vi "Read 1 Swipe X Z Vector.vi"(8 "Error In":errorcluster, 11 "Leap Handle":T2) -> (0 "Error Out":errorcluster, 1 "Gesture State":T1, 2 "XZ Swipe Vector":cluster{"X Direction":sgl, "Z Direction":sgl}, 3 "Leap Handle":T2)   [LabVIEW 2011, in "LVH-Leap.lvlib"]
uses:
  LVH-Leap.lvlib
  Private/Type Defs/Leap Handle.ctl
  C:/github/labviewhacker/LVH-Leap/LabVIEW/vi.lib/LabVIEW Hacker/Leap/Private/Libs/LeapCSharp.NET3.5.dll
  Private/Libs/LeapCSharp.NET3.5.dll
  Private/Type Defs/Gesture State.ctl
  Read 1 Swipe.vi
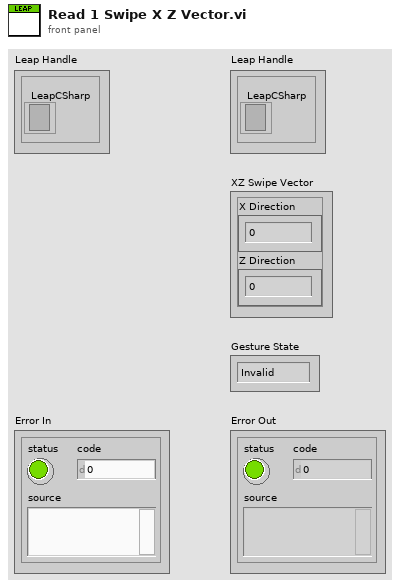
[diagram p1: front panel]
types:
  T1 = typedef "LVH-Leap.lvlib/Gesture State.ctl" = enum16{"Invalid", "Start", "Update", "Stop"}
  T2 = typedef "LVH-Leap.lvlib/Leap Handle.ctl" = cluster{"LeapCSharp":refnum<k24>}
  T3 = typedef "LVH-Leap.lvlib/Gesture Swipe.ctl" = cluster{"Common":T4, "Direction":T6, "Position":T6, "Start Position":T6, "Speed":dbl}
  T4 = typedef "LVH-Leap.lvlib/Gesture Common.ctl" = cluster{"ID":dbl, "Duration (S)":dbl, "Gesture Type":T5, "Gesture State":T1}
  T5 = typedef "LVH-Leap.lvlib/Gesture Type.ctl" = enum16{"Invalid", "Swipe", "Circle", "Screen Tap", "Key Tap"}
  T6 = typedef "LVH-Leap.lvlib/Vector.ctl" = cluster{"Pitch":sgl, "Yaw":sgl, "Roll":sgl, "Magnitude":sgl, "XYZ":sgl[]}
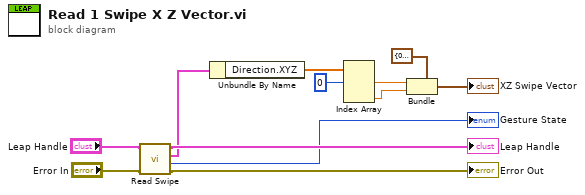
[diagram p0: block diagram]
diagram:
  n1 = call-poly "Read Swipe.vi"("Error In"="Error In", "Leap Handle"="Leap Handle") -> ("Error Out"=→"Error Out":errorcluster, "Swipe Status"=→"Gesture State":T1, "Swipe"=w2:T3, "Leap Handle"=→"Leap Handle":T2)  [unwired: 6 in]
  n2 = Unbundle By Name(w2) -> ("Direction.XYZ"=w10:sgl[])
  n3 = Index Array(array=w10, index #1=0 ("index")) -> (element #1=w11:sgl, element #3=w9:sgl)  [unwired: 2 in, 1 out]
  n4 = Bundle(cluster=cluster{"X Direction":sgl, "Z Direction":sgl} {"X Direction"=0.0, "Z Direction"=0.0} ("element"), "X Direction"=w11, "Z Direction"=w9) -> (→"XZ Swipe Vector":cluster{"X Direction":sgl, "Z Direction":sgl})
